vi "Generate Arguments.vi"(7 "command is subsystem":bool, 8 "error in (no error)":errorcluster, 9 "command":string, 11 "client in":refnum<class "PuTTY Client.lvclass">) -> (0 "error out":errorcluster, 2 "arguments":string[](array[string]), 3 "client out":refnum<class "PuTTY Client.lvclass">, 5 "environment variables":cluster{"name":string, "value":string}[](array[cluster]))   [LabVIEW 2020, in "NI_SSH.lvlib" / "PuTTY Client.lvclass"]
uses:
  <vilib>/net/SSH/Client/PuTTY/PuTTY Client.lvclass
  e:/builds/penguin/labview/branches/2020/dev/dist/vi.lib/net/SSH/Client/Generic/Generic Client.lvclass
  <vilib>/net/SSH/Client/PuTTY/PuTTY Client.lvclass/PuTTY Client.ctl
  <vilib>/net/SSH/Client/Generic/Generic Client.lvclass/Generic Client.ctl
  <vilib>/net/SSH/Client/Generic/Read identity.vi
  <vilib>/net/SSH/Client/Generic/Read user_host.vi
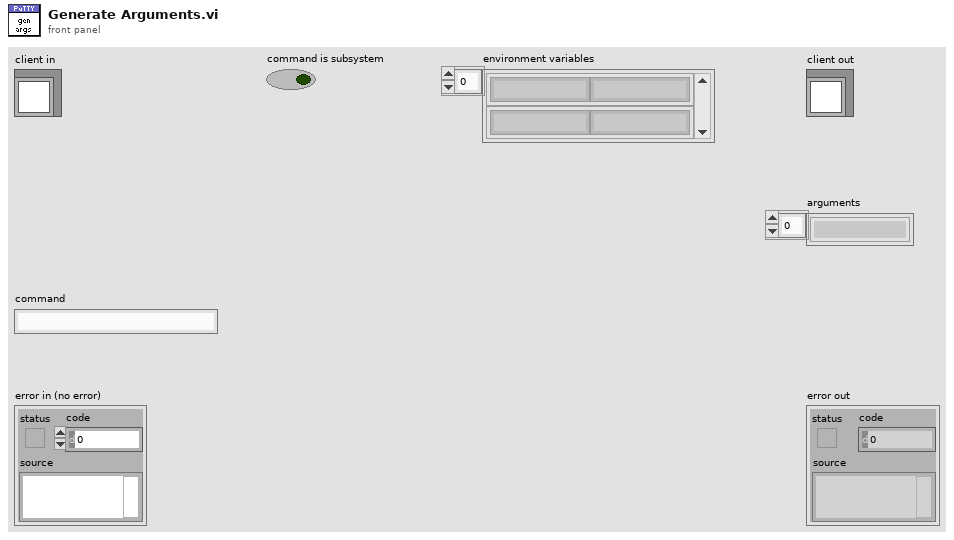
[diagram p1: front panel]
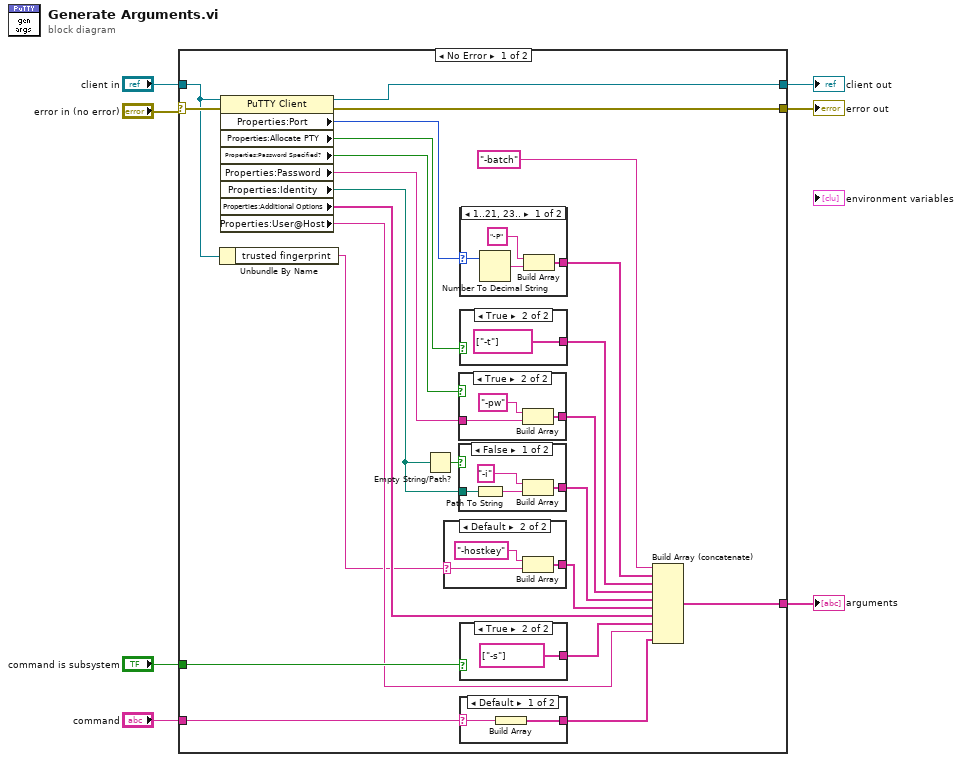
[diagram p0: block diagram]
diagram:
  n1 = case shown="No Error" "error in (no error)" {
    selector: "error in (no error)" -> [w25 w50]
    tunnel: "client in" -> [w10 w51]
    tunnel: "command is subsystem" -> [w24 _]
    tunnel: "command" -> [w22 _]
    tunnel: [w20 _] -> w3
    tunnel: [w19 w51] -> w2
    tunnel: [w18 w50] -> w1
    frame No Error {
      n2 = Unbundle By Name(w10) -> ("trusted fingerprint"=w9:string)
      n3 = property on="Property Node" class="PuTTY Client"(reference=w10, error in=w25) -> (reference out=w19:refnum<class "PuTTY Client.lvclass">, error out=w18:errorcluster, "Properties:Port"=w31:u16, "Properties:Allocate PTY"=w30:bool, "Properties:Password Specified?"=w17:bool, "Properties:Password"=w16:string, "Properties:Identity"=w13:path, "Properties:Additional Options"=w26:string[], "Properties:User@Host"=w11:string)
      n4 = Empty String/Path?(string/path=w13) -> (empty?=w14:bool)
      n5 = case shown="Default" w9 {
        selector: w9 -> [_ w32]
        tunnel: [_ w33] -> w8
        frame "" {
        }
        frame Default {
          n6 = Build Array("-hostkey", w32) -> (w33:string[])
        }
      }
      n7 = case shown="True" w17 {
        tunnel: w16 -> [_ w43]
        tunnel: [_ w42] -> w15
        frame False {
        }
        frame True {
          n8 = Build Array("-pw", w43) -> (w42:string[])
        }
      }
      n9 = case shown="False" w14 {
        tunnel: w13 -> [w36 _]
        tunnel: [w37 _] -> w12
        frame False {
          n10 = Path To String(path=w36) -> (string=w35:string)
          n11 = Build Array("-i", w35) -> (w37:string[])
        }
        frame True {
        }
      }
      n12 = case shown="1..21, 23.." w31 {
        selector: w31 -> [w47 _]
        tunnel: [w49 _] -> w28
        frame 1..21, 23.. {
          n13 = Number To Decimal String(number=w47) -> (decimal integer string=w46:string)  [unwired: 1 in]
          n14 = Build Array("-P", w46) -> (w49:string[])
        }
        frame ..0, 22 {
        }
      }
      n15 = case shown="True" w30 {
        tunnel: [_ string[] ["-t"]] -> w27
        frame False {
        }
        frame True {
        }
      }
      n16 = case shown="True" w24 {
        tunnel: [_ string[] ["-s"]] -> w23
        frame False {
        }
        frame True {
        }
      }
      n17 = case shown="Default" w22 {
        selector: w22 -> [w40 _]
        tunnel: [w39 _] -> w21
        frame Default {
          n18 = Build Array(w40) -> (w39:string[])
        }
        frame "" {
        }
      }
      n19 = Build Array (concatenate)("-batch", w28, w27, w15, w12, w8, w26, w23, w11, w21) -> (w20:string[])
    }
    frame Error {
    }
  }
  "error out" <- w1
  "client out" <- w2
  "arguments" <- w3
